vi "Принтер.vi"() -> ()   [LabVIEW 2021]
uses:
  Control.ctl
  Control 5.ctl
  Control 4.ctl
panel:
  out "Сообщение":string
  out "Ингредиенты":T1
  out "СТакан":T2 scale=0.0..200.0
  in  "Молоко":dbl(slide) scale=0.0..1000.0
  in  "Вода":dbl(slide) scale=0.0..3000.0
  in  "Кофе":dbl(slide) scale=0.0..1000.0
  in  "Меню":T3
  in  "stop":bool
  out "Состояние":T4
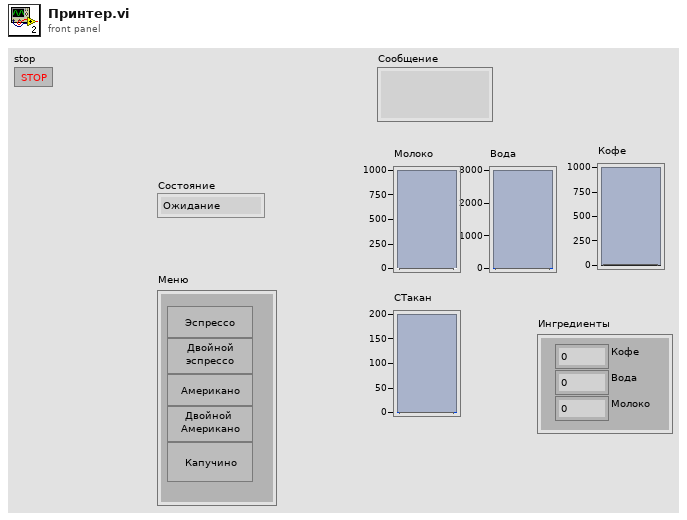
[diagram p1: front panel]
types:
  T1 = typedef "Control 4.ctl" = cluster{"Кофе":dbl, "Вода":dbl, "Молоко":dbl}
  T2 = typedef "Control 5.ctl" = dbl
  T3 = typedef "Кофе.ctl" = cluster{"Эспрессо":bool, "Двойной\nэспрессо":bool, "Американо":bool, "Двойной \nАмерикано":bool, "Капучино":bool}
  T4 = typedef "Control.ctl" = enum16{"Ожидание", "Выбор пользователя", "Анализ ошибок", "Анализ", "Перемол Кофе", "Добавь воды", "Добавь молоко", "Заберите стакан"}
  T5 = enum8{"Enabled", "Disabled", "Disabled and Grayed Out"}
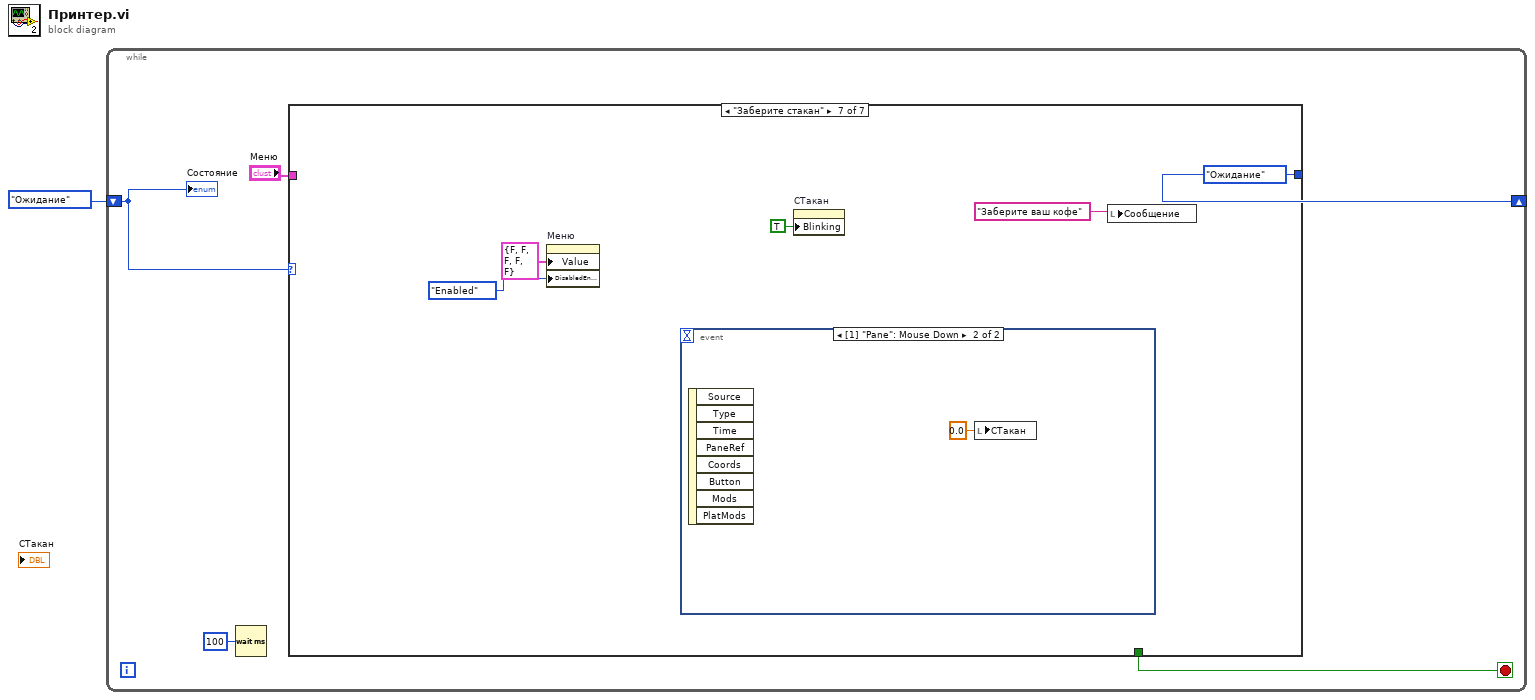
[diagram p0: block diagram]
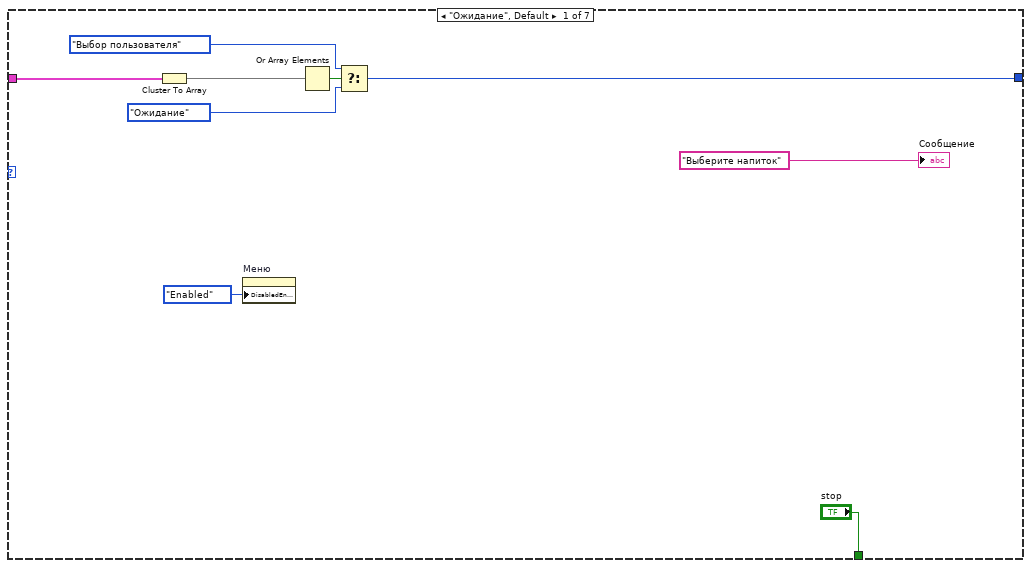
[diagram p2: hidden frame]
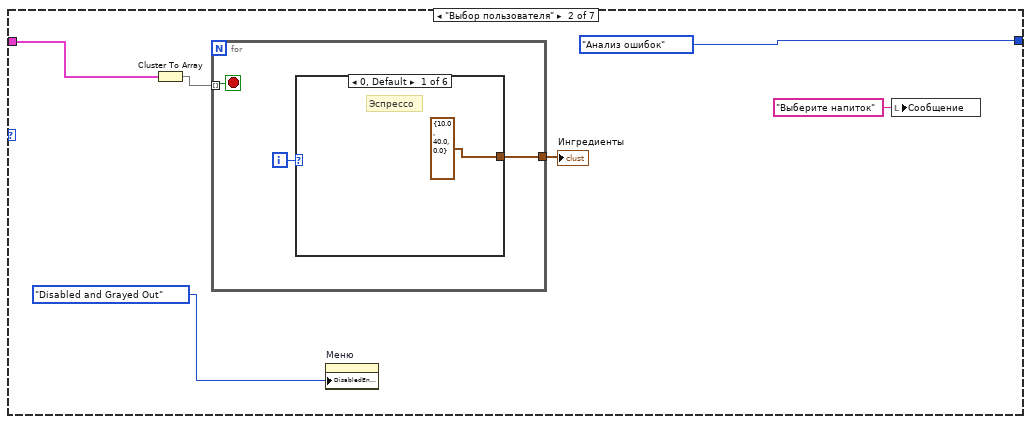
[diagram p3: hidden frame]
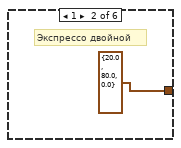
[diagram p4: hidden frame]
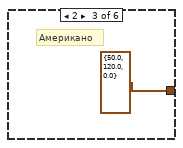
[diagram p5: hidden frame]
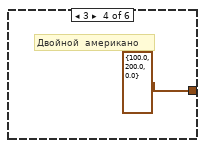
[diagram p6: hidden frame]
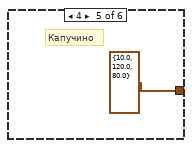
[diagram p7: hidden frame]
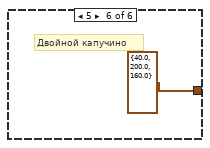
[diagram p8: hidden frame]
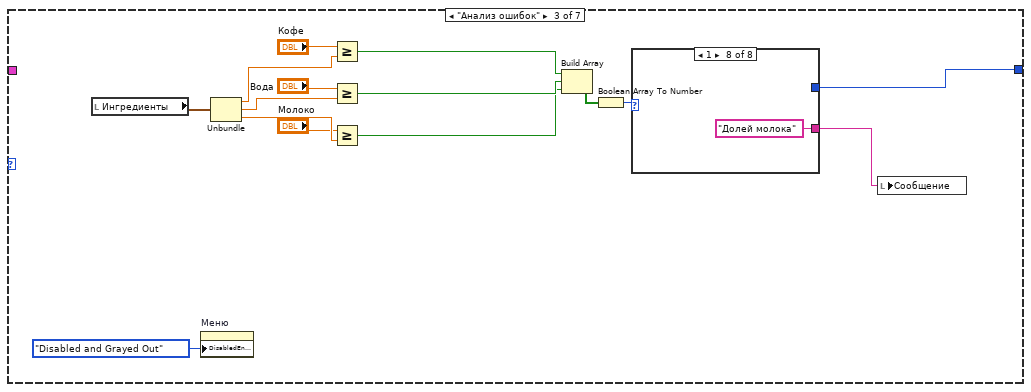
[diagram p9: hidden frame]
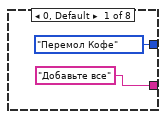
[diagram p10: hidden frame]
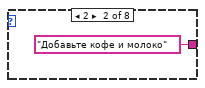
[diagram p11: hidden frame]
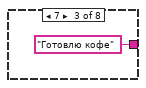
[diagram p12: hidden frame]
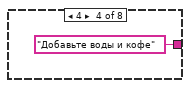
[diagram p13: hidden frame]
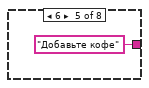
[diagram p14: hidden frame]
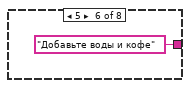
[diagram p15: hidden frame]
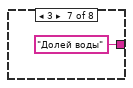
[diagram p16: hidden frame]
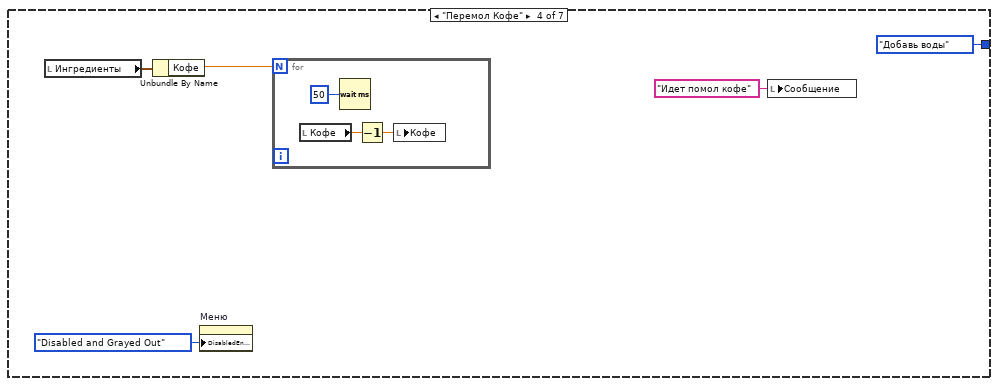
[diagram p17: hidden frame]
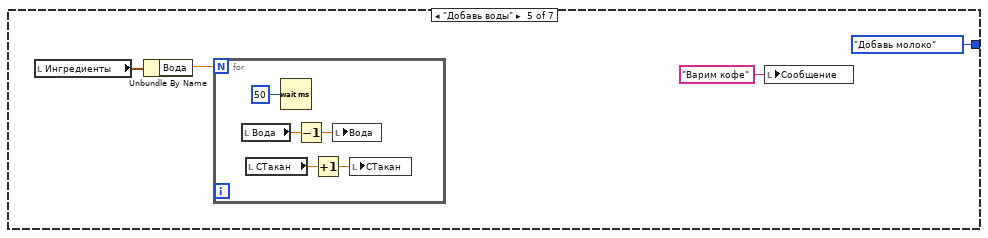
[diagram p18: hidden frame]
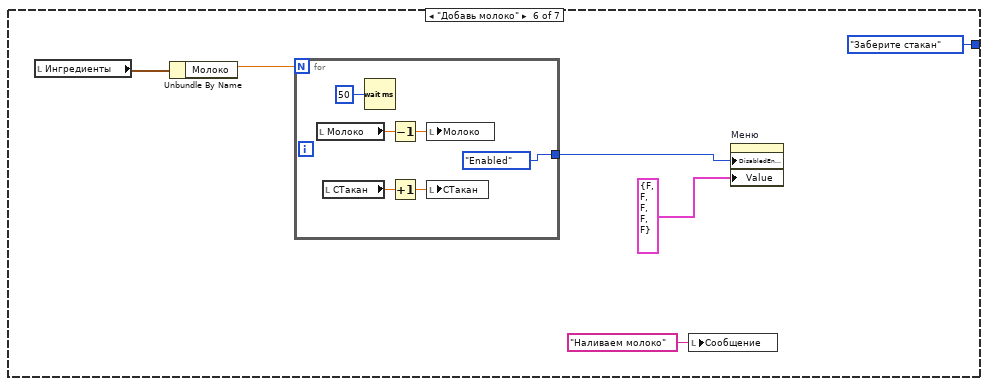
[diagram p19: hidden frame]
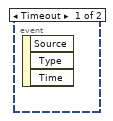
[diagram p20: hidden frame]
diagram:
  n1 = while {
    shift-right: [w2] -> _
    shift-left: Control."Ожидание" ("Enum") -> [w6]
    stop <- w5 stop-if-true
    n2 = Wait (ms)(milliseconds to wait=u32 100) -> ()  [unwired: 1 out]
    n3 = case shown="\"Заберите стакан\"" w6 {
      tunnel: ["stop" _ _ _ _ _ _] -> w5
      tunnel: "Меню" -> [w13 w21 _ _ _ _ _]
      tunnel: [w9 Control."Анализ ошибок" ("Enum") w33 Control."Добавь воды" ("Enum") Control."Добавь молоко" ("Enum") Control."Заберите стакан" ("Enum") Control."Ожидание" ("Enum")] -> w2
      frame "Ожидание", Default {
        n4 = Cluster To Array(cluster=w13) -> (array=w14:bool[])
        n5 = property on="Меню" class="Clust (strict)"("DisabledEnum"=T5."Enabled" ("Disabled")) -> ()  [unwired: 2 in, 2 out]
        n6 = Or Array Elements(Boolean array=w14) -> (logical OR=w12:bool)
        n7 = Select(t=Control."Выбор пользователя" ("Enum"), s=w12, f=Control."Ожидание" ("Enum")) -> (s? t:f=w9:T4)
        "Сообщение" <- "Выберите напиток"
      }
      frame "Выбор пользователя" {
        n8 = Cluster To Array(cluster=w21) -> (array=w20:bool[])
        n9 = for {
          tunnel: w20 -> [w24] mode=indexing
          tunnel: [w22] -> w18
          i -> [w23]
          stop <- w24 stop-if-true
          n10 = case shown="0, Default" w23 {
            tunnel: [T1 {"Кофе"=10.0, "Вода"=40.0, "Молоко"=0.0} ("Ингредиенты") T1 {"Кофе"=20.0, "Вода"=80.0, "Молоко"=0.0} ("Ингредиенты") T1 {"Кофе"=50.0, "Вода"=120.0, "Молоко"=0.0} ("Ингредиенты") T1 {"Кофе"=100.0, "Вода"=200.0, "Молоко"=0.0} ("Ингредиенты") T1 {"Кофе"=10.0, "Вода"=120.0, "Молоко"=80.0} ("Ингредиенты") T1 {"Кофе"=40.0, "Вода"=200.0, "Молоко"=160.0} ("Ингредиенты")] -> w22
            frame 0, Default {
              # "Эспрессо"
            }
            frame 1 {
              # "Экспрессо двойной"
            }
            frame 2 {
              # "Американо"
            }
            frame 3 {
              # "Двойной  американо"
            }
            frame 4 {
              # "Капучино"
            }
            frame 5 {
              # "Двойной капучино"
            }
          }
        }
        "Ингредиенты" <- w18
        n11 = property on="Меню" class="Clust (strict)"("DisabledEnum"=T5."Disabled and Grayed Out" ("Disabled")) -> ()  [unwired: 2 in, 2 out]
        n12 = local write "Сообщение"("Выберите напиток" ("Сообщение")) -> ()
      }
      frame "Анализ ошибок" {
        n13 = local read "Ингредиенты"() -> (w45:T1)
        n14 = property on="Меню" class="Clust (strict)"("DisabledEnum"=T5."Disabled and Grayed Out" ("Disabled")) -> ()  [unwired: 2 in, 2 out]
        n15 = Unbundle(w45) -> ("Кофе"=w42:dbl, "Вода"=w43:dbl, "Молоко"=w44:dbl)
        n16 = Greater Or Equal?(x="Кофе", y=w42) -> (x >= y?=w38:bool)
        n17 = Greater Or Equal?(x="Вода", y=w43) -> (x >= y?=w37:bool)
        n18 = Greater Or Equal?(x="Молоко", y=w44) -> (x >= y?=w36:bool)
        n19 = Build Array(w38, w37, w36) -> (w34:bool[])
        n20 = Boolean Array To Number(Boolean array=w34) -> (number=w35:u32)
        n21 = case shown="1" w35 {
          tunnel: ["Добавьте все" "Добавьте кофе и молоко" "Готовлю кофе" "Добавьте воды и кофе" "Добавьте кофе" "Добавьте воды и кофе" "Долей воды" "Долей молока"] -> w31
          tunnel: [Control."Перемол Кофе" ("Enum") _ _ _ _ _ _ _] -> w33
          frame 0, Default {
          }
          frame 2 {
          }
          frame 7 {
          }
          frame 4 {
          }
          frame 6 {
          }
          frame 5 {
          }
          frame 3 {
          }
          frame 1 {
          }
        }
        n22 = local write "Сообщение"(w31) -> ()
      }
      frame "Перемол Кофе" {
        n23 = local read "Ингредиенты"() -> (w59:T1)
        n24 = Unbundle By Name(w59) -> ("Кофе"=w58:dbl)
        n25 = property on="Меню" class="Clust (strict)"("DisabledEnum"=T5."Disabled and Grayed Out" ("Disabled")) -> ()  [unwired: 2 in, 2 out]
        n26 = for {
          N: w58 -> [_]
          n27 = local read "Кофе"() -> (w60:dbl)
          n28 = Wait (ms)(milliseconds to wait=u32 50) -> ()  [unwired: 1 out]
          n29 = Decrement(x=w60) -> (x-1=w61:dbl)
          n30 = local write "Кофе"(w61) -> ()
        }
        n31 = local write "Сообщение"("Идет помол кофе") -> ()
      }
      frame "Добавь воды" {
        n32 = local read "Ингредиенты"() -> (w66:T1)
        n33 = Unbundle By Name(w66) -> ("Вода"=w65:dbl)
        n34 = for {
          N: w65 -> [_]
          n35 = local read "Вода"() -> (w69:dbl)
          n36 = local read "СТакан"() -> (w67:T2)
          n37 = Wait (ms)(milliseconds to wait=u32 50) -> ()  [unwired: 1 out]
          n38 = Decrement(x=w69) -> (x-1=w70:dbl)
          n39 = Increment(x=w67) -> (x+1=w68:T2)
          n40 = local write "Вода"(w70) -> ()
          n41 = local write "СТакан"(w68) -> ()
        }
        n42 = local write "Сообщение"("Варим кофе") -> ()
      }
      frame "Добавь молоко" {
        n43 = local read "Ингредиенты"() -> (w77:T1)
        n44 = Unbundle By Name(w77) -> ("Молоко"=w76:dbl)
        n45 = for {
          N: w76 -> [_]
          tunnel: [T5."Enabled" ("Disabled")] -> w74
          n46 = local read "Молоко"() -> (w82:dbl)
          n47 = local read "СТакан"() -> (w79:T2)
          n48 = Wait (ms)(milliseconds to wait=u32 50) -> ()  [unwired: 1 out]
          n49 = Decrement(x=w82) -> (x-1=w81:dbl)
          n50 = Increment(x=w79) -> (x+1=w80:T2)
          n51 = local write "Молоко"(w81) -> ()
          n52 = local write "СТакан"(w80) -> ()
        }
        n53 = local write "Сообщение"("Наливаем молоко") -> ()
        n54 = property on="Меню" class="Clust (strict)"("DisabledEnum"=w74, "Value"=T3 {"Эспрессо"=FALSE, "Двойной\nэспрессо"=FALSE, "Американо"=FALSE, "Двойной \nАмерикано"=FALSE, "Капучино"=FALSE}) -> ()  [unwired: 2 in, 2 out]
      }
      frame "Заберите стакан" {
        n55 = property on="Меню" class="Clust (strict)"("Value"=T3 {"Эспрессо"=FALSE, "Двойной\nэспрессо"=FALSE, "Американо"=FALSE, "Двойной \nАмерикано"=FALSE, "Капучино"=FALSE} ("Меню"), "DisabledEnum"=T5."Enabled" ("Disabled")) -> ()  [unwired: 2 in, 2 out]
        n56 = event shown="[1] \"Pane\": Mouse Down" {
          selector: _ -> [_ _]
          dyn-events: _ -> [_ _]
          timeout: _ -> [_ _]
          event Timeout {
            n57 = event-data() -> ()  [unwired: 1 in, 3 out]
          }
          event Mouse Down {
            n58 = event-data() -> ()  [unwired: 1 in, 8 out]
            n59 = local write "СТакан"(T2 0.0 ("СТакан")) -> ()
          }
        }
        n60 = property on="СТакан" class="Slide (strict)"("Blinking"=TRUE) -> ()  [unwired: 2 in, 2 out]
        n61 = local write "Сообщение"("Заберите ваш кофе") -> ()
      }
    }
    "Состояние" <- w6
  }
